vi "Stop Core.vi"(10 "final error code":i32, 11 "tWorkerController in":refnum<class "tWorkerController.lvclass">) -> (3 "tWorkerController out":refnum<class "tWorkerController.lvclass">)   [LabVIEW 2013, in "tWorkerController.lvlib" / "tWorkerController.lvclass"]
doc: "(<B>Filename</B>: Actor Framework.lvlib:Actor.lvclass:Stop Core.vi)\n\nDefines what the actor does before it stops. Use the <B>final error code</B> input to determine whether the actor shut down in response to an error.\n\nBy default, this method does nothing. A descendant class may override it to define behavior, such as shutting down any processes the actor initiated in its override of the Actor Core method."
uses:
  tWorkerController.lvclass
  <vilib>/ActorFramework/Actor/Actor.lvclass
  tWorkerController.lvclass/tWorkerController.ctl
  <vilib>/ActorFramework/Message Enqueuer/Message Enqueuer.lvclass/Message Enqueuer.ctl
  <vilib>/ActorFramework/Message Enqueuer/Enqueue.vi
  <vilib>/ActorFramework/Message Priority Queue/Priority Enqueue.vi
  tWorkerTCPConnection/msgs/Quit Msg/Quit Msg.lvclass
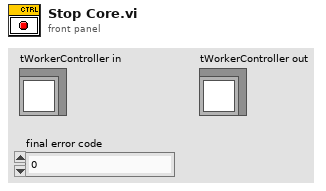
[diagram p1: front panel]
types:
  T1 = typedef "tWorkerController.lvlib/tWorkerController.lvclass/_tcpConnection.ctl" = cluster{"GUID":string, "Connection Queue":refnum<class "Message Enqueuer.lvclass">, "PID":i64}
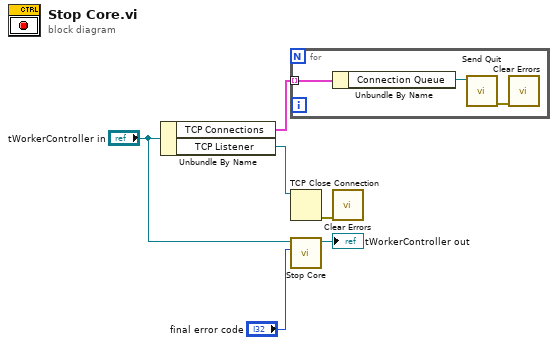
[diagram p0: block diagram]
diagram:
  n1 = Unbundle By Name("tWorkerController in") -> ("TCP Connections"=w4:T1[], "TCP Listener"=w3:refnum<k5>)
  n2 = for {
    tunnel: w4 -> [w9] mode=indexing
    n3 = Unbundle By Name(w9) -> ("Connection Queue"=w8:refnum<class "Message Enqueuer.lvclass">)
    n4 = call "Send Quit.vi"("Message Enqueuer"=w8) -> ("error out"=w7:errorcluster)  [unwired: 9 in, 1 out]
    n5 = call <vilib>:"Clear Errors.vi"("error in (no error)"=w7) -> ()  [unwired: 6 in, 1 out]
  }
  n6 = TCP Close Connection(connection ID=w3) -> (error out=w2:errorcluster)  [unwired: 2 in, 1 out]
  n7 = call-parent "Stop Core.vi"("final error code"="final error code", "Actor in"="tWorkerController in") -> ("Actor out"=→"tWorkerController out":refnum<class "tWorkerController.lvclass">)  [unwired: 9 in]
  n8 = call <vilib>:"Clear Errors.vi"("error in (no error)"=w2) -> ()  [unwired: 6 in, 1 out]
